vi "IsMessageRegistered.vi"(8 "error in (no error)":errorcluster, 11 "SendMessage in":refnum<class "SendMessage.lvclass">) -> (0 "error out":errorcluster, 1 "Message Que is Registered":bool, 3 "SendMessage out":refnum<class "SendMessage.lvclass">)   [LabVIEW 2019, in "SendMessage.lvclass"]
uses:
  SendMessage.lvclass
  SendMessage.lvclass/SendMessage.ctl
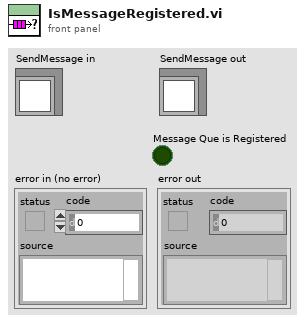
[diagram p1: front panel]
types:
  T1 = typedef "MessageQue.lvlib/MessageQue.ctl" = refnum<queue>
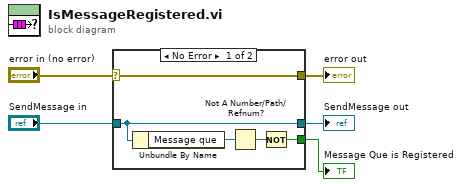
[diagram p0: block diagram]
diagram:
  n1 = case shown="No Error" "error in (no error)" {
    selector: "error in (no error)" -> [w10 w12]
    tunnel: [w10 w12] -> w4
    tunnel: [w9 w11] -> w2
    tunnel: "SendMessage in" -> [w9 w11]
    tunnel: [w6 _] -> w1
    frame No Error {
      n2 = Unbundle By Name(w9) -> ("Message que"=w8:T1)
      n3 = Not A Number/Path/Refnum?(number/path/refnum=w8) -> (NaN/Path/Refnum?=w7:bool)
      n4 = Not(x=w7) -> (.not. x?=w6:bool)
    }
    frame Error {
    }
  }
  "error out" <- w4
  "SendMessage out" <- w2
  "Message Que is Registered" <- w1
